vi "WPILogGetEntryCount.vi"(8 "error in (no error)":errorcluster, 11 "Data Value Reference in":refnum<data-value>) -> (0 "error out":errorcluster, 3 "Entires":i32)   [LabVIEW 2020]
uses:
  Typedef/WPILibLog.ctl
  Typedef/Header.ctl
  Typedef/Entry.ctl
  Typedef/Record.ctl
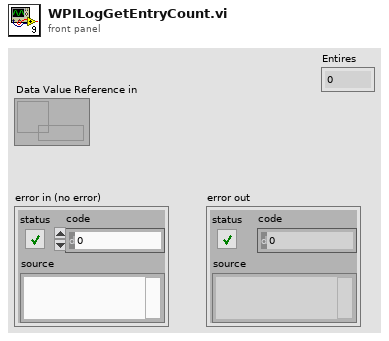
[diagram p1: front panel]
types:
  T1 = typedef "WPILibLog.ctl" = cluster{"Header":T2, "Record Start Idx":i32, "Entries":map{u32, T3}, "file ref":refnum<file>, "Finished Entries":T3[], "raw data":u8[]}
  T2 = typedef "Header.ctl" = cluster{"Header String":string, "Version":dbl, "Header Extra String Length":u32, "Header Extra String":string}
  T3 = typedef "Entry.ctl" = cluster{"ID":u32, "Records":T4[], "Finished?":bool, "Name":string, "Type":string, "Metadata":string, "RecordCnt":i32}
  T4 = typedef "Record.ctl" = cluster{"raw data":u8[], "ID":u32, "Size (bytes)":u32, "Timestamp":u64}
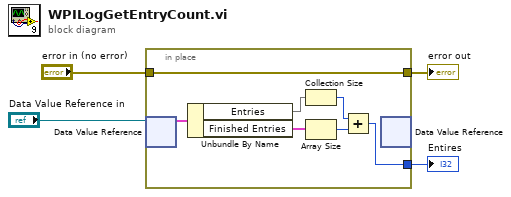
[diagram p0: block diagram]
diagram:
  n1 = in-place {
    in-place-border: "error in (no error)" -> [w6]
    in-place-border: [w6] -> w4
    in-place-border: [w5] -> w1
    n2 = in-place-dvr #1("Data Value Reference in") -> (w11:T1)  [unwired: 1 out]
    n3 = Unbundle By Name(w11) -> ("Entries"=w10:map{u32, T3}, "Finished Entries"=w7:T3[])
    n4 = Collection Size(1:w10) -> (0:w9:i32)
    n5 = Array Size(array=w7) -> (size(s)=w8:i32)
    n6 = Add(x=w9, y=w8) -> (x+y=w5:i32)
    n7 = in-place-dvr #1() -> ()  [unwired: 1 in, 2 out]
  }
  "error out" <- w4
  "Entires" <- w1
